vi "Create DblMessage.vi"(8 "error in (no error)":errorcluster, 10 "Message Data":dbl, 11 "Message Name":string) -> (0 "error out":errorcluster, 3 "DblMessage Out":refnum<class "DblMessage.lvclass">)   [LabVIEW 2009, in "LapDog.Messaging.v2.NativeTypes.lvlib" / "DblMessage.lvclass"]
doc: "Returns a DblMessage object with the given name.\n\nThis method executes regardless of the error in state."
uses:
  DblMessage.lvclass
  DblMessage.lvclass/DblMessage.ctl
  Messaging.v2/MessageObject/Message.lvclass
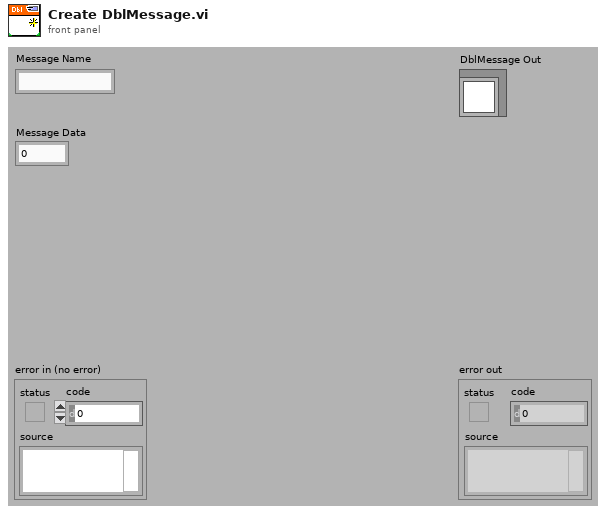
[diagram p1: front panel]
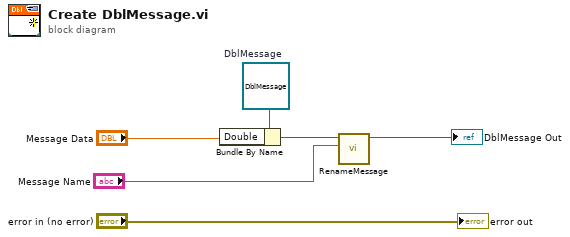
[diagram p0: block diagram]
diagram:
  w6 = refnum<class "DblMessage.lvclass"> refnum  # DblMessage
  n1 = Bundle By Name(cluster=w6, "Double"="Message Data") -> (w3:refnum<class "DblMessage.lvclass">)
  n2 = call "RenameMessage.vi"("Message Name"="Message Name", "Message in"=w3) -> ("Message out"=→"DblMessage Out":refnum<class "DblMessage.lvclass">)  [unwired: 8 in, 1 out]
  "error out" <- "error in (no error)"
